vi "Syringe Config to Inner Area Register Data.vi"(0 "Syringe Configuration":T1={"Syringe Speicification"=1.0, "Volume Unit"=1, "Syringe Length"=57.1513, "Syringe Length Unit"=0} caption="注射器配置" {"Syringe Length Unit" items=["mm"]; "Syringe Length" min=0.001; "Volume Unit" items=["mL"=1, "uL"=2]; "Syringe Speicification" min=0.001}) -> (7 "Valid Result":bool caption="有效结果", 9 "Value Reg Data":dbl caption="值寄存器", 10 "Unit Reg Data":dbl caption="单位寄存器")   [LabVIEW 2023, in "Longer Pump dLSP501 Series.lvlib"]
uses:
  <instrlib>/Longer Pump dLSP501 Modbus RTU Series/Longer Pump dLSP501 Series.lvlib
panel:
  # "缺省定义：\ndLSP501W: 规格 1mL, 行程 57.1513mm"
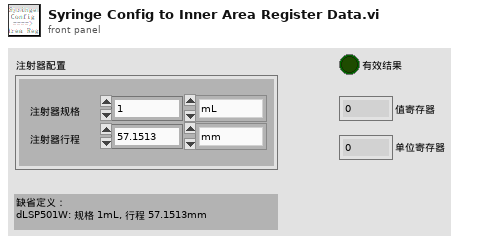
[diagram p1: front panel]
types:
  T1 = cluster{"Syringe Speicification":dbl, "Volume Unit":u16, "Syringe Length":dbl, "Syringe Length Unit":u16}
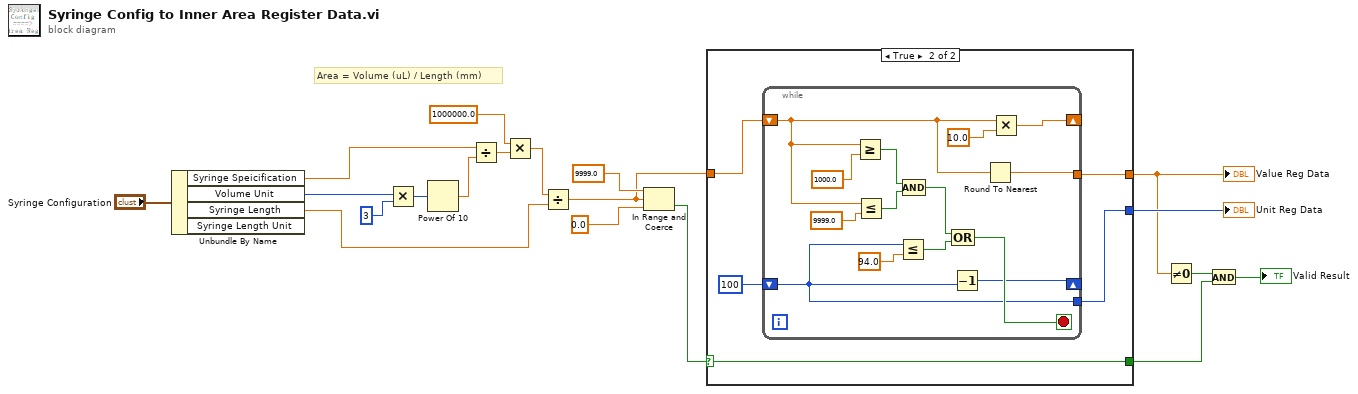
[diagram p0: block diagram]
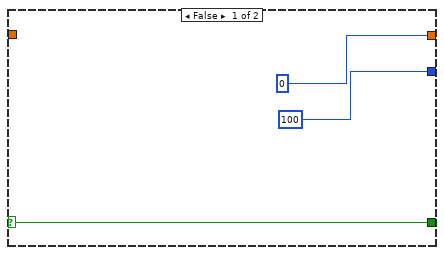
[diagram p2: hidden frame]
diagram:
  # "Area = Volume (uL) / Length (mm)"
  n1 = Unbundle By Name("Syringe Configuration") -> ("Syringe Speicification"=w9:dbl, "Volume Unit"=w4:u16, "Syringe Length"=w8:dbl)  [unwired: 1 out]
  n2 = Multiply(x=w4, y=u16 3) -> (x*y=w6:u16)
  n3 = Power Of 10(x=w6) -> (10^x=w5:dbl)
  n4 = Divide(x=w9, y=w5) -> (x/y=w2:dbl)
  n5 = Multiply(x=1000000.0 ("y"), y=w2) -> (x*y=w3:dbl)
  n6 = Divide(x=w3, y=w8) -> (x/y=w16:dbl)
  n7 = In Range and Coerce(upper limit=9999.0 ("x"), x=w16, lower limit=0.0 ("x")) -> (In Range?=w17:bool)  [unwired: 1 out]
  n8 = case shown="True" w17 {
    selector: w17 -> [w22 w27]
    tunnel: w16 -> [_ w26]
    tunnel: [w22 w27] -> w11
    tunnel: [100 w23] -> w15
    tunnel: [0 w24] -> w13
    frame False {
    }
    frame True {
      n9 = while {
        shift-right: [w41] -> _
        shift-left: w26 -> [w29]
        shift-right: [w32] -> _
        shift-left: 100 -> [w30]
        tunnel: [w28] -> w24
        tunnel: [w30] -> w23
        stop <- w34 stop-if-true
        n10 = Greater Or Equal?(x=w29, y=1000.0 ("x")) -> (x >= y?=w37:bool)
        n11 = Less Or Equal?(x=w29, y=9999.0 ("x")) -> (x <= y?=w36:bool)
        n12 = Less Or Equal?(x=w30, y=94.0 ("x")) -> (x <= y?=w31:bool)
        n13 = Compound Arithmetic op=AND ("复合运算")(w37, w36) -> (w35:bool)
        n14 = Compound Arithmetic op=OR ("复合运算")(w35, w31) -> (w34:bool)
        n15 = Decrement(x=w30) -> (x-1=w32:i32)
        n16 = Round To Nearest(number=w29) -> (nearest integer value=w28:dbl)
        n17 = Multiply(x=w29, y=10.0) -> (x*y=w41:dbl)
      }
    }
  }
  "Value Reg Data" <- w13
  "Unit Reg Data" <- w15
  n18 = Not Equal To 0?(x=w13) -> (x != 0?=w14:bool)
  n19 = And(x=w14, y=w11) -> (x .and. y?=→"Valid Result":bool)
